vi "header_in.vi"(10 "HEADER":string) -> (2 "FINS Header":T1={"resp req"=FALSE, "cmd resp"=FALSE, "SID"=255, "DNA"=2, "DA1"=2, "DA2"=2, "SA1"=0, "SA2"=255, "SNA"=255} {"SNA" max=127 format="%x"; "SA2" max=254 step=1 format="%x"; "SA1" format="%x"; "DA2" max=254 step=1 format="%x"; "DA1" format="%x"; "DNA" max=127 step=1 format="%x"})   [LabVIEW 2020, in "FINS TCP.lvlib"]
uses:
  FINS TCP.lvlib
  FINS_header.ctl
panel:
  out "Barray":u8[](array[numeric]) format="%x"
  # "hex"
  # "1.ICS"
  # "2.RSV"
  # "3.GCT"
  # "4.DNA"
  # "5.DA1"
  # "6.DA2"
  # "7.SNA"
  # "8.SA1_node"
  # "9.SA1_unit"
  # "10.SID"
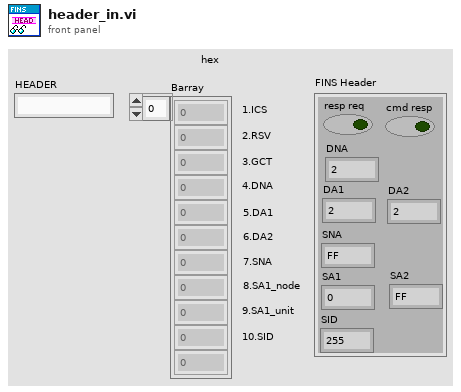
[diagram p1: front panel]
types:
  T1 = typedef "FINS TCP.lvlib/FINS_header.ctl" = cluster{"resp req":bool, "cmd resp":bool, "SID":u8, "DNA":u8, "DA1":u8, "DA2":u8, "SA1":u8, "SA2":u8, "SNA":u8}
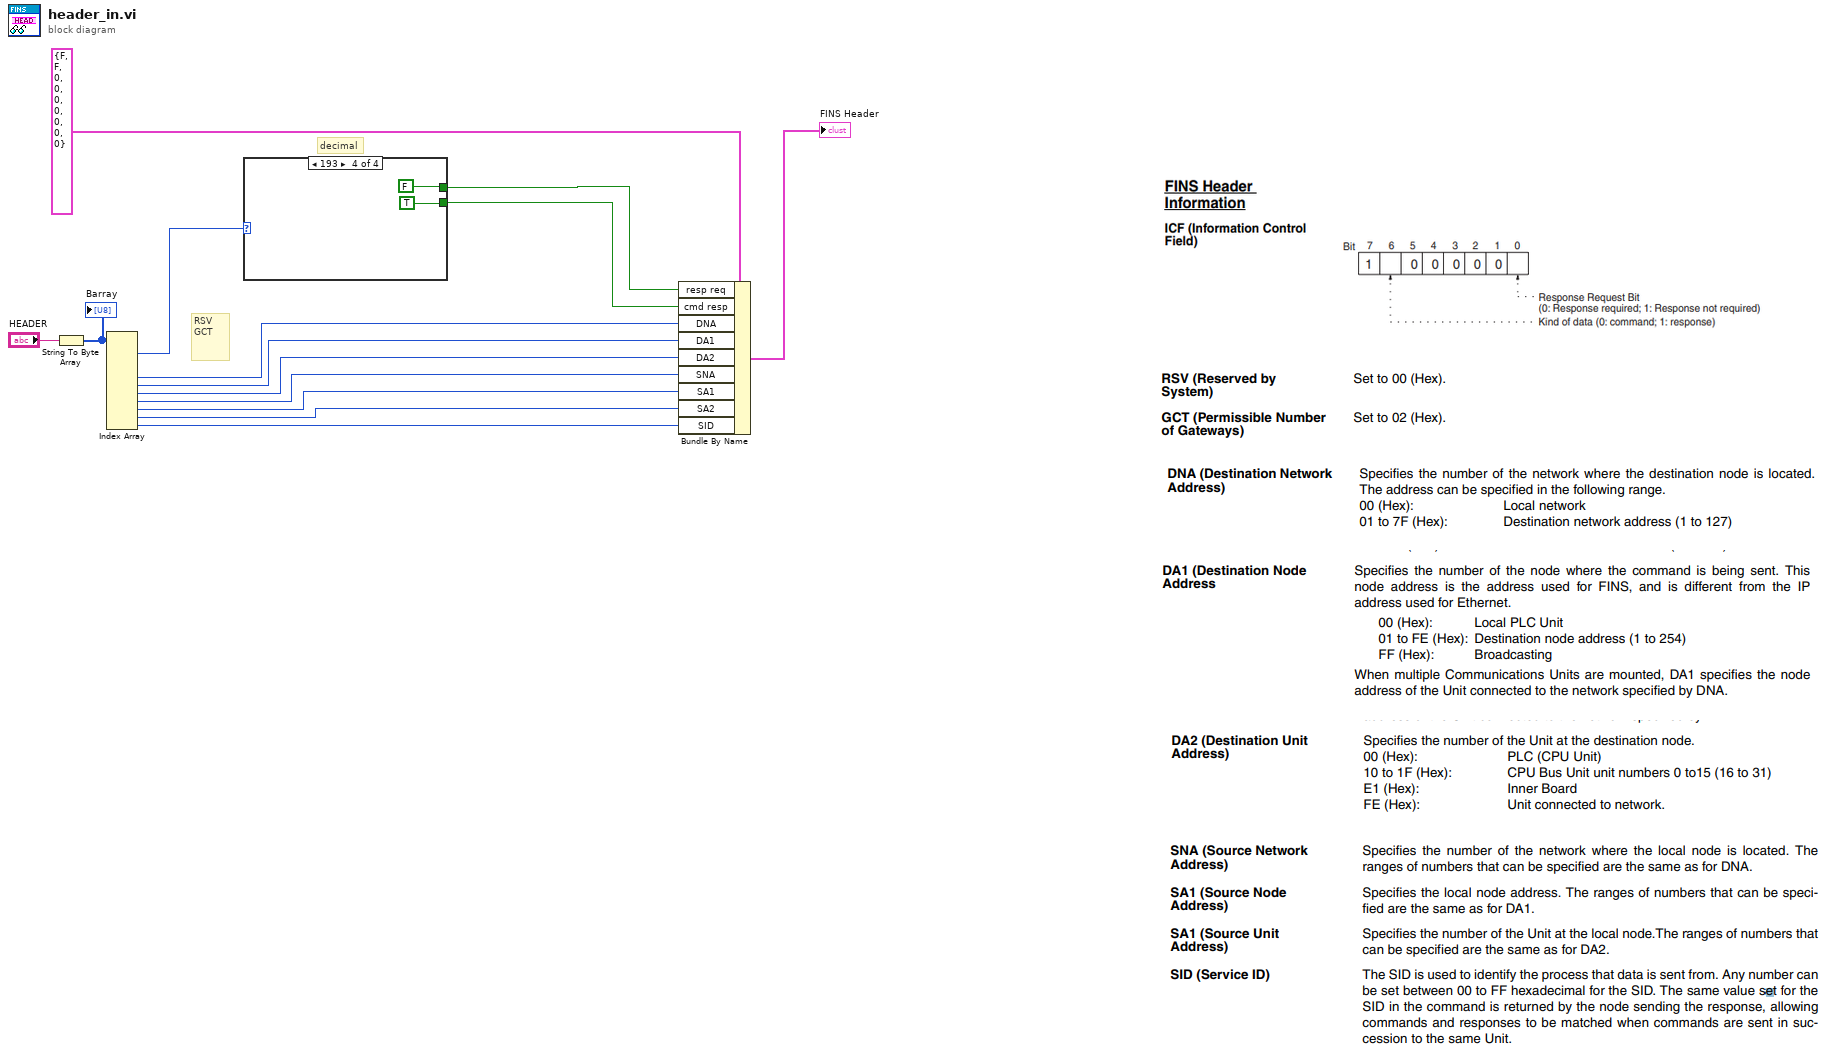
[diagram p0: block diagram]
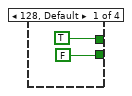
[diagram p2: hidden frame]
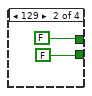
[diagram p3: hidden frame]
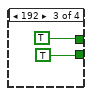
[diagram p4: hidden frame]
diagram:
  # "decimal"
  # "RSV\nGCT"
  n1 = String To Byte Array(string="HEADER") -> (unsigned byte array=w14:u8[])
  "Barray" <- w14
  n2 = Index Array(array=w14) -> (element #1=w1:u8, element #4=w8:u8, element #5=w7:u8, element #6=w6:u8, element #7=w5:u8, element #8=w4:u8, element #9=w3:u8, element #10=w2:u8)  [unwired: 10 in, 2 out]
  n3 = case shown="193" w1 {
    tunnel: [TRUE FALSE TRUE FALSE] -> w11
    tunnel: [FALSE FALSE TRUE TRUE] -> w10
    frame 128, Default {
    }
    frame 129 {
    }
    frame 192 {
    }
    frame 193 {
    }
  }
  n4 = Bundle By Name(cluster=T1 {"resp req"=FALSE, "cmd resp"=FALSE, "SID"=0, "DNA"=0, "DA1"=0, "DA2"=0, "SA1"=0, "SA2"=0, "SNA"=0} ("FINS Header 2"), "resp req"=w11, "cmd resp"=w10, "DNA"=w8, "DA1"=w7, "DA2"=w6, "SNA"=w5, "SA1"=w4, "SA2"=w3, "SID"=w2) -> (→"FINS Header":T1)
